vi "Set Time Scale.vi"(8 "TRIARC_ERROR_IN":errorcluster, 10 "Time Scale [ms]":u32, 11 "Person In":refnum<class "Person.lvclass">) -> (0 "TRIARC_ERROR_OUT":errorcluster, 3 "Person Out":refnum<class "Person.lvclass">)   [LabVIEW 2020, in "Person.lvclass"]
uses:
  Person.lvclass
  Person.lvclass/Person.ctl
  <vilib>/Astemes/Triarc Framework/Process/Process.lvclass
  C:/Program Files (x86)/National Instruments/LabVIEW 2020/vi.lib/Astemes/Triarc Framework/View/View.lvclass
  C:/Program Files (x86)/National Instruments/LabVIEW 2020/vi.lib/Astemes/Triarc Framework/Process/Process.lvclass
  C:/Program Files (x86)/National Instruments/LabVIEW 2020/vi.lib/Astemes/Triarc Framework/Base/Base.lvclass
  C:/Program Files (x86)/National Instruments/LabVIEW 2020/vi.lib/Astemes/Triarc Framework/Error Handler Interface/Error Handler Interface.lvclass
  C:/Program Files (x86)/National Instruments/LabVIEW 2020/vi.lib/Astemes/Triarc Framework/Logging/Logging.lvclass
  C:/git/astemes-triarc-examples/source/Coffee Shop/Processes/People/Person/Person.lvclass
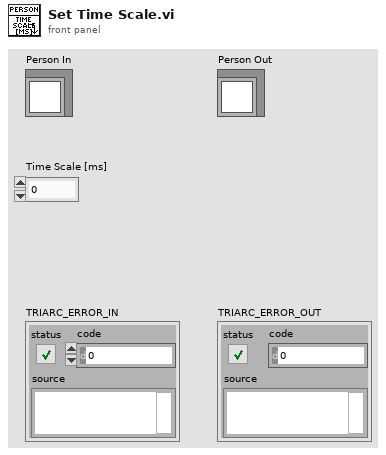
[diagram p1: front panel]
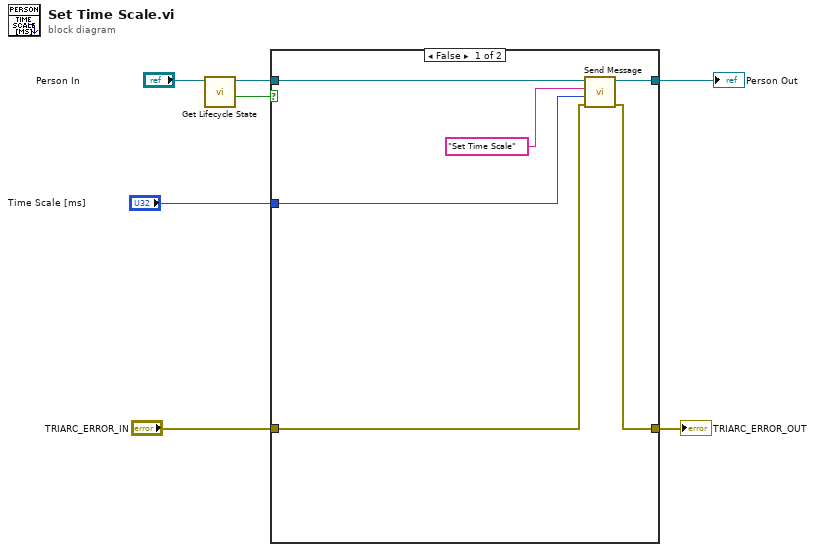
[diagram p0: block diagram]
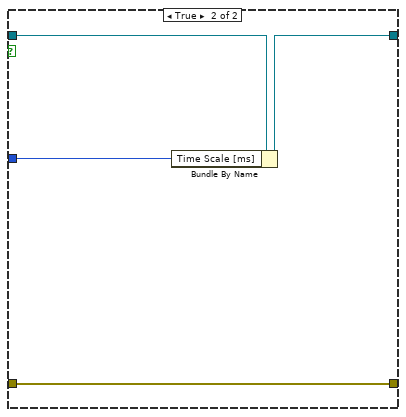
[diagram p2: hidden frame]
diagram:
  n1 = call <vilib>:"Get Lifecycle State.vi"("Process In"="Person In") -> ("In Process Loop?"=w3:bool, "Process Out"=w6:refnum<class "Person.lvclass">)  [unwired: 7 in, 2 out]
  n2 = case shown="False" w3 {
    tunnel: w6 -> [w13 w17]
    tunnel: [w12 w15] -> w5
    tunnel: "TRIARC_ERROR_IN" -> [w8 w16]
    tunnel: [w9 w16] -> w4
    tunnel: "Time Scale [ms]" -> [w11 w14]
    frame False {
      n3 = call <vilib>:"Send Message.vi"("error in (no error)"=w8, "Message Data"=w11, "Message"="Set Time Scale" ("API Message"), "Process In"=w13) -> ("error out"=w9:errorcluster, "Process Out"=w12:refnum<class "Person.lvclass">)  [unwired: 6 in]
    }
    frame True {
      n4 = Bundle By Name(cluster=w17, "Time Scale [ms]"=w14) -> (w15:refnum<class "Person.lvclass">)
    }
  }
  "TRIARC_ERROR_OUT" <- w4
  "Person Out" <- w5
